vi "TargetAngle.vi"(1 "Horizontal_Pixel":dbl) -> (0 "TargetAngle":dbl)   [LabVIEW 2015]
panel:
  # "in degrees"
  # "Made by Matt Carr\non 8 Febuary 2016"
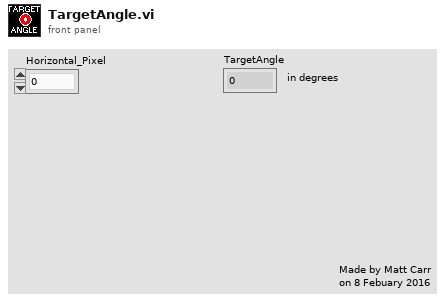
[diagram p1: front panel]
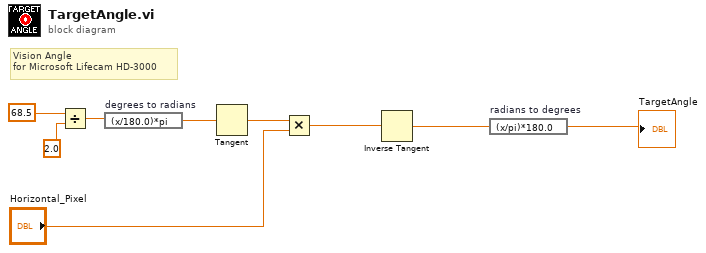
[diagram p0: block diagram]
diagram:
  # "Vision Angle\nfor Microsoft Lifecam HD-3000"
  n1 = Divide(x=68.5, y=2.0) -> (x/y=w7:dbl)
  n2 = expression code="(x/180.0)*pi" "degrees to radians"(w7) -> (w6:dbl)
  n3 = Tangent(1:w6) -> (0:w5:dbl)
  n4 = Multiply(x=w5, y="Horizontal_Pixel") -> (x*y=w3:dbl)
  n5 = Inverse Tangent(1:w3) -> (0:w2:dbl)
  n6 = expression code="(x/pi)*180.0" "radians to degrees"(w2) -> (→"TargetAngle":dbl)
